vi "Initalize.vi"(8 "error in (no error)":errorcluster, 11 "Instruments in":refnum<class "Instruments.lvclass">) -> (0 "error out":errorcluster, 3 "Instruments out":refnum<class "Instruments.lvclass">)   [LabVIEW 2012, in "Instruments.lvclass"]
uses:
  Instruments.lvclass
  Instruments.lvclass/Instruments.ctl
panel:
  out "Ophir Board":string
  out "Debug Index":i32
  in  "integration time (medium:1)":u16(ring)=1 items=["fast perod", "medium period", "line cycle period @ 50Hz", "line cycle period @ 60Hz"]
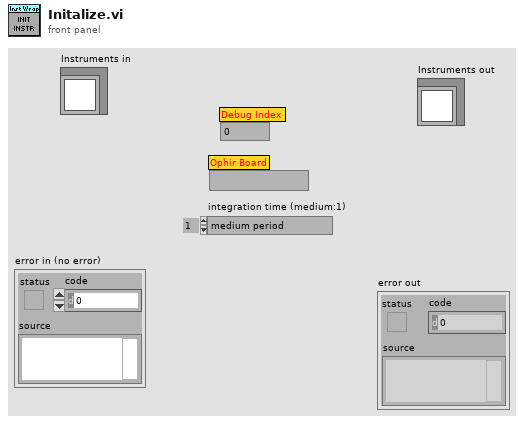
[diagram p1: front panel]
types:
  T1 = typedef "USB4000_Data.ctl" = cluster{"Wrapper Out":u32, "Number of Spectrometers":i32, "Wavelength":dbl[], "EL Spectrum":dbl[], "Int Time (usec)":i32, bool, "Background":dbl[]}
  T2 = cluster{"Keithley_Param":cluster{"Start Current,mA":dbl, "Stop Current,mA":dbl, "Voltage Compliance,V":dbl, "GPIB":string}, "USB4000_Param":cluster{"Integration Time":i32, "Wl min,nm":dbl, "Wl max,nm":dbl, "USB4000":T1}, "Ophir_Param":cluster{"VISA resource name":refnum<visa-resource-name>, "Calibration Wl":dbl}}
  T3 = cluster{"Start Current,mA":dbl, "Stop Current,mA":dbl, "Voltage Compliance,V":dbl, "GPIB":string}
  T4 = cluster{"Integration Time":i32, "Wl min,nm":dbl, "Wl max,nm":dbl, "USB4000":T1}
  T5 = cluster{"error":bool, "code":i32, "source":string}
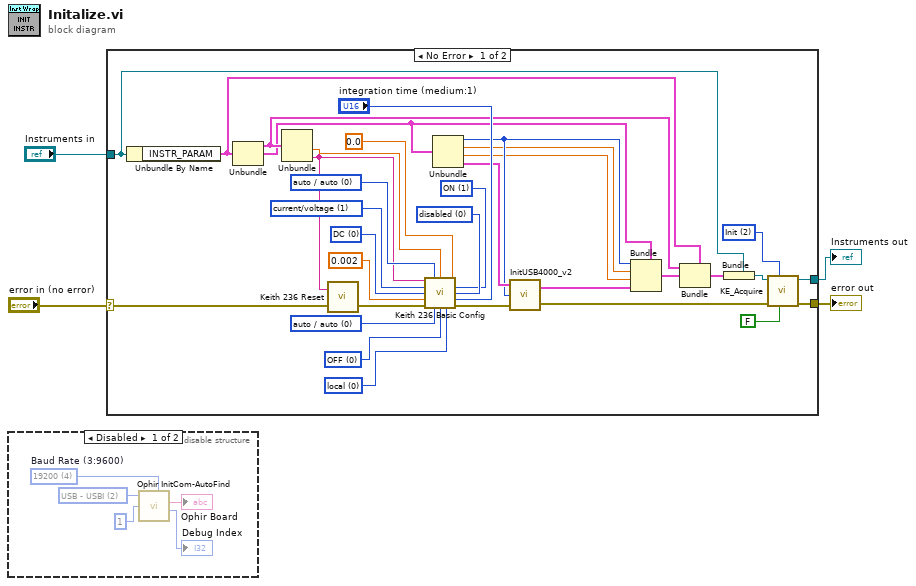
[diagram p0: block diagram]
diagram:
  n1 = disable-structure shown="Disabled" {
    frame Disabled {
      w7 = i16 4 items=["300", "1200", "4800", "9600", "19200", "38400"]  # Baud Rate (3:9600)
      w5 = i16 2 items=["USB - Nova2", "USB - Vega", "USB - USBI", "RS232", "GPIB"] ("communication")
      n2 = call "Ophir InitCom-AutoFind.vi"("Baud Rate (3:9600)"=w7, "communication"=w5, "Port Number (default 2)"=i16 1) -> ("Ophir Board"=→"Ophir Board":string, "Debug Index"=→"Debug Index":i32)  [unwired: 1 in, 2 out]
    }
    frame Enabled {
    }
  }
  n3 = case shown="No Error" "error in (no error)" {
    selector: "error in (no error)" -> [w20 w44]
    tunnel: [w11 w44] -> w3
    tunnel: [w14 w43] -> w1
    tunnel: "Instruments in" -> [w22 w43]
    frame No Error {
      w12 = u16 2 items=["First", "Second", "Init"] ("Type")
      w33 = u16 1 items=["OFF", "ON"] ("default delay (on:1)")
      w34 = u16 0 items=["disabled", "2 readings", "4 readings", "8 readings", "16 readings", "32 readings"] ("filter (disabled:0)")
      w36 = u16 0 items=["local", "remote"] ("sense (local:0)")
      w37 = u16 0 items=["OFF", "ON"] ("suppression (off:0)")
      w38 = u16 0 items=["auto / auto", "1 nA / 1.1 V", "10 nA / 11 V", "100 nA / 110 V", "0.001 mA / 110 V", "0.01 mA / 110 V", "0.1 mA / 110 V", "1 mA / 110 V", "10 mA / 110 V", "100 mA / 110 V"] ("compliance/\nmeasurement range (auto:0)")
      w39 = u16 0 items=["DC", "sweep"] ("function (DC:0)")
      w40 = u16 1 items=["voltage/current", "current/voltage"] ("source/measure (V/I:0)")
      w42 = u16 0 items=["auto / auto", "1 nA / 1.1 V", "10 nA / 11 V", "100 nA / 110 V", "0.001 mA / 110 V", "0.01 mA / 110 V", "0.1 mA / 110 V", "1 mA / 110 V", "10 mA / 110 V", "100 mA / 110 V"] ("source range\nI source / V source (auto:0)")
      n4 = Unbundle By Name(w22) -> ("INSTR_PARAM"=w23:T2)
      n5 = Unbundle(w23) -> ("Keithley_Param"=w28:T3, "USB4000_Param"=w26:T4)  [unwired: 1 out]
      n6 = Unbundle(w28) -> ("Voltage Compliance,V"=w30:dbl, "GPIB"=w29:string)  [unwired: 2 out]
      n7 = call "Keith 236 Reset.vi"("GPIB address"=w29, "error in"=w20) -> ("error out"=w41:T5)
      n8 = call "Keith 236 Basic Config.vi"("GPIB address"=w29, "source range\nI source / V source (auto:0)"=w42, "voltage \ncompliance level"=w30, "DC delay (sec)"=0.0, "source/measure (V/I:0)"=w40, "default delay (on:1)"=w33, "function (DC:0)"=w39, "filter (disabled:0)"=w34, "source level"=0.002, "integration time (medium:1)"="integration time (medium:1)", "error in"=w41, "compliance/\nmeasurement range (auto:0)"=w38, "suppression (off:0)"=w37, "sense (local:0)"=w36) -> ("error out"=w31:T5)  [unwired: 1 in]
      n9 = Unbundle(w26) -> ("Integration Time"=w19:i32, "Wl min,nm"=w18:dbl, "Wl max,nm"=w17:dbl, "USB4000"=w27:T1)
      n10 = call "InitUSB4000_v2.vi"("error in (no error)"=w31, "Int Time (usec)"=w19, "USB4000 In"=w27) -> ("error out"=w10:errorcluster, "USB4000 Out"=w25:T1)
      n11 = Bundle(cluster=w26, "Integration Time"=w19, "Wl min,nm"=w18, "Wl max,nm"=w17, "USB4000"=w25) -> (w24:T4)
      n12 = Bundle(cluster=w23, "Keithley_Param"=w28, "USB4000_Param"=w24) -> (w21:T2)  [unwired: 1 in]
      n13 = Bundle(cluster=w22, w21) -> (w15:refnum<class "Instruments.lvclass">)
      n14 = call-dynamic "KE_Acquire.vi"("Boolean"=FALSE, "Type"=w12, "error in (no error)"=w10, "Instruments in"=w15) -> ("error out"=w11:errorcluster, "Instruments out"=w14:refnum<class "Instruments.lvclass">)  [unwired: 5 in, 1 out]
    }
    frame Error {
    }
  }
  "error out" <- w3
  "Instruments out" <- w1
